vi "owl actions.vi"(6 "OWL parameters":T2={"T (sec)"=1.2701010101010102, "owl?"=enum."focus", "A (rad)"=1.2701010101010102, "refit ?"=enum."refit"} {"T (sec)" scale=1.0..20.0; "A (rad)" scale=0.1..1.57}, 7 "owl action":T1, 9 "delta phase (rad) IN":dbl=289.5873590533738, 11 "time in (sec)":dbl=289.5873590533738) -> (0 "phase (rad) OUT":dbl=289.5873590533738, 1 "delta phase (rad) OUT":dbl=289.5873590533738)   [LabVIEW 2020]
uses:
  owl parameters.ctl
  owl action.ctl
  owl -- send for fit action.ctl
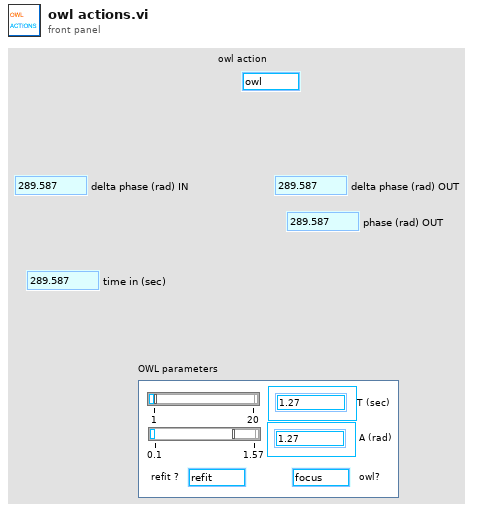
[diagram p1: front panel]
types:
  T1 = typedef "owl action.ctl" = enum16{"owl", "focus"}
  T2 = typedef "owl parameters.ctl" = cluster{"T (sec)":dbl, "owl?":T1, "A (rad)":dbl, "refit ?":T3}
  T3 = typedef "owl -- send for fit action.ctl" = enum16{"refit", "chill"}
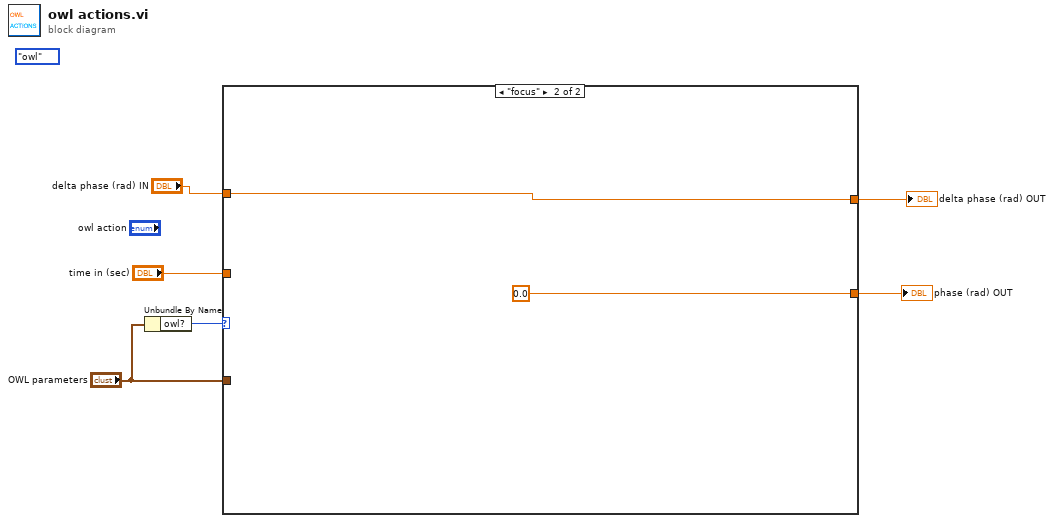
[diagram p0: block diagram]
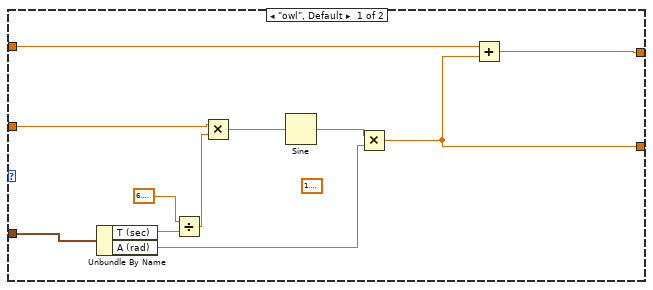
[diagram p2: hidden frame]
diagram:
  (unwired) owl_action."owl" ("owl action")
  n1 = Unbundle By Name("OWL parameters") -> ("owl?"=w2:T1)
  n2 = case shown="\"focus\"" w2 {
    tunnel: [w9 w19] -> w6
    tunnel: "time in (sec)" -> [w17 _]
    tunnel: "OWL parameters" -> [w16 _]
    tunnel: "delta phase (rad) IN" -> [w10 w19]
    tunnel: [w7 0.0 ("phase (rad) OUT")] -> w1
    frame "owl", Default {
      (unwired) 1.5707963267948966
      n3 = Unbundle By Name(w16) -> ("T (sec)"=w14:dbl, "A (rad)"=w8:dbl)
      n4 = Divide(x=6.283185307179586, y=w14) -> (x/y=w13:dbl)
      n5 = Multiply(x=w17, y=w13) -> (x*y=w12:dbl)
      n6 = Sine(x=w12) -> (sin(x)=w11:dbl)
      n7 = Multiply(x=w11, y=w8) -> (x*y=w7:dbl)
      n8 = Add(x=w10, y=w7) -> (x+y=w9:dbl)
    }
    frame "focus" {
    }
  }
  "delta phase (rad) OUT" <- w6
  "phase (rad) OUT" <- w1
